vi "hax.vi"(11 "string":string) -> (3 "output cluster":T1)   [LabVIEW 2014]
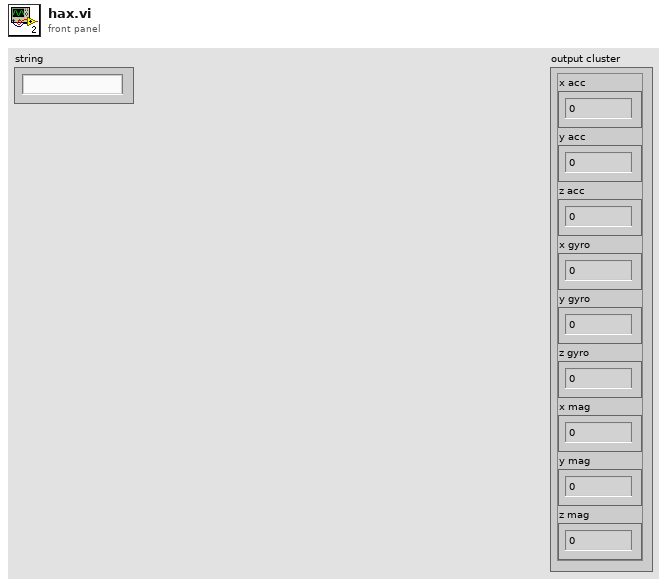
[diagram p1: front panel]
types:
  T1 = cluster{"x acc":i16, "y acc":i16, "z acc":i16, "x gyro":i16, "y gyro":i16, "z gyro":i16, "x mag":i16, "y mag":i16, "z mag":i16}
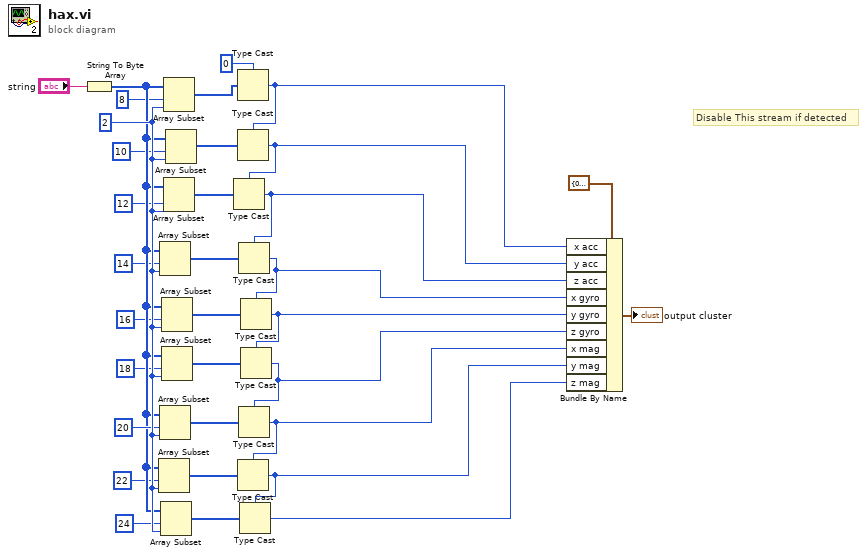
[diagram p0: block diagram]
diagram:
  w24 = 2 ("length")
  # "Disable This stream if detected"
  n1 = String To Byte Array(string="string") -> (unsigned byte array=w22:u8[])
  n2 = Array Subset(array=w22, index=22, length=w24) -> (w17:u8[])
  n3 = Array Subset(array=w22, index=14, length=w24) -> (w6:u8[])
  n4 = Array Subset(array=w22, index=20, length=w24) -> (w21:u8[])
  n5 = Array Subset(array=w22, index=24, length=w24) -> (w20:u8[])
  n6 = Array Subset(array=w22, index=16, length=w24) -> (w13:u8[])
  n7 = Array Subset(array=w22, index=18, length=w24) -> (w16:u8[])
  n8 = Array Subset(array=w22, index=8, length=w24) -> (w11:u8[])
  n9 = Array Subset(array=w22, index=12, length=w24) -> (w5:u8[])
  n10 = Array Subset(array=w22, index=10, length=w24) -> (w12:u8[])
  n11 = Type Cast(type=i16 0, x=w11) -> (*(type *) &x=w25:i16)
  n12 = Type Cast(type=w25, x=w12) -> (*(type *) &x=w26:i16)
  n13 = Type Cast(type=w26, x=w5) -> (*(type *) &x=w27:i16)
  n14 = Type Cast(type=w27, x=w6) -> (*(type *) &x=w33:i16)
  n15 = Type Cast(type=w33, x=w13) -> (*(type *) &x=w28:i16)
  n16 = Type Cast(type=w28, x=w16) -> (*(type *) &x=w29:i16)
  n17 = Type Cast(type=w29, x=w21) -> (*(type *) &x=w30:i16)
  n18 = Type Cast(type=w30, x=w17) -> (*(type *) &x=w31:i16)
  n19 = Type Cast(type=w31, x=w20) -> (*(type *) &x=w32:i16)
  n20 = Bundle By Name(cluster=T1 {"x acc"=0, "y acc"=0, "z acc"=0, "x gyro"=0, "y gyro"=0, "z gyro"=0, "x mag"=0, "y mag"=0, "z mag"=0} ("Raw IMU"), "x acc"=w25, "y acc"=w26, "z acc"=w27, "x gyro"=w33, "y gyro"=w28, "z gyro"=w29, "x mag"=w30, "y mag"=w31, "z mag"=w32) -> (→"output cluster":T1)
